vi "PlayMP3.vi"(8 "Error In":errorcluster, 11 "Path":path) -> (0 "Error out":errorcluster)   [LabVIEW 2021]
doc: "Play mp3 file from given path."
uses:
  04a88a2a-43ca-4840-871c-c4acfed5d58f.vi
panel:
  in  "WindowsMediaPlayer":refnum<k7>(container)
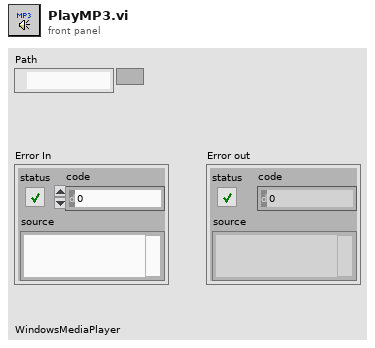
[diagram p1: front panel]
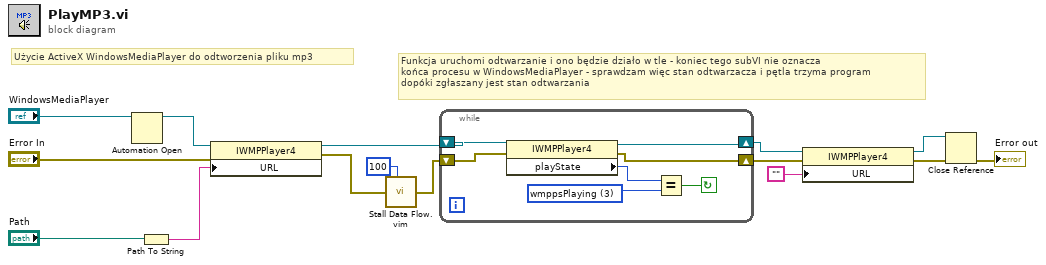
[diagram p0: block diagram]
diagram:
  # "Funkcja uruchomi odtwarzanie i ono będzie działo w tle - koniec tego subVI nie oznacza\nkońca procesu w WindowsMediaPlayer - sprawdzam więc stan odtwarzacza i pętla trzyma program \ndopóki zgłaszany jest stan odtwarzania"
  # "Użycie ActiveX WindowsMediaPlayer do odtworzenia pliku mp3"
  n1 = Automation Open(Automation Refnum="WindowsMediaPlayer") -> (Automation Refnum=w14:refnum<k7>)  [unwired: 1 in, 3 out]
  n2 = Path To String(path="Path") -> (string=w13:string)
  n3 = property class="IWMPPlayer4"(reference=w14, error in="Error In", "URL"=w13) -> (reference out=w9:refnum<k7>, error out=w12:errorcluster)
  n4 = call "Stall Data Flow.vim"("value in"=w12, "milliseconds to wait"=u32 100) -> ("value out"=w8:errorcluster)  [unwired: 1 out]
  n5 = while {
    shift-right: [w21] -> w10
    shift-left: w8 -> [w22]
    shift-right: [w19] -> w5
    shift-left: w9 -> [w20]
    stop <- w16 continue-if-true
    w17 = 3 items=["wmppsUndefined", "wmppsStopped", "wmppsPaused", "wmppsPlaying", "wmppsScanForward", "wmppsScanReverse", "wmppsBuffering", "wmppsWaiting", "wmppsMediaEnded", "wmppsTransitioning", "wmppsReady", "wmppsReconnecting", "wmppsLast"] ("playState 2")
    n6 = property class="IWMPPlayer4"(reference=w20, error in=w22) -> (reference out=w19:refnum<k7>, error out=w21:errorcluster, "playState"=w18:i32)
    n7 = Equal?(x=w18, y=w17) -> (x = y?=w16:bool)
  }
  n8 = property class="IWMPPlayer4"(reference=w5, error in=w10, "URL"="") -> (reference out=w4:refnum<k7>, error out=w6:errorcluster)
  n9 = Close Reference(reference=w4, error in (no error)=w6) -> (error out=→"Error out":errorcluster)
